vi "Activity Log.vi"(6 "Log File Path":path, 7 "Action":T1, 8 "Error In":errorcluster, 9 "string ref":refnum<vi>, 11 "Message Log Entry":string) -> (0 "Error Out":errorcluster, 3 "Message Log":string)   [LabVIEW 2024]
doc: "This functional global timestamps and records text messages for a generic message log."
uses:
  Activity Log enum Action .ctl
panel:
  in  "Max Lines":i32=8000
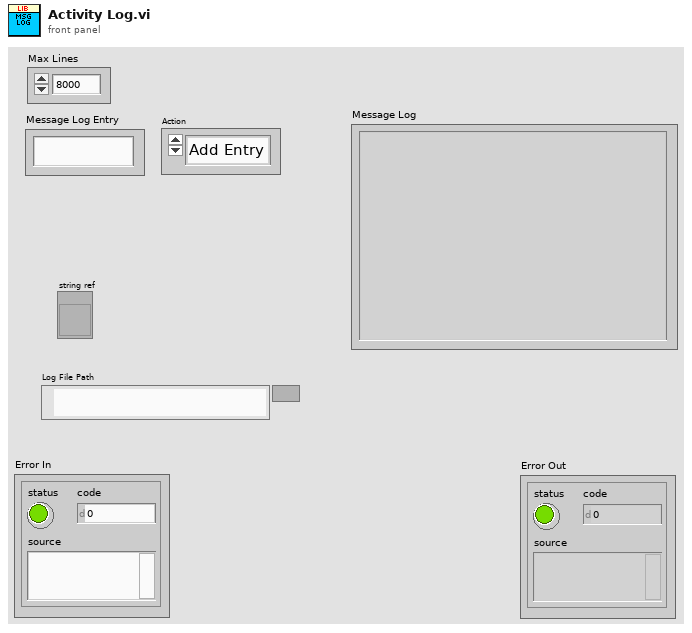
[diagram p1: front panel]
types:
  T1 = typedef "Activity Log enum Action .ctl" = enum16{"Add Entry", "Get Log", "Restore From Disk", "Save to Disk", "Init"}
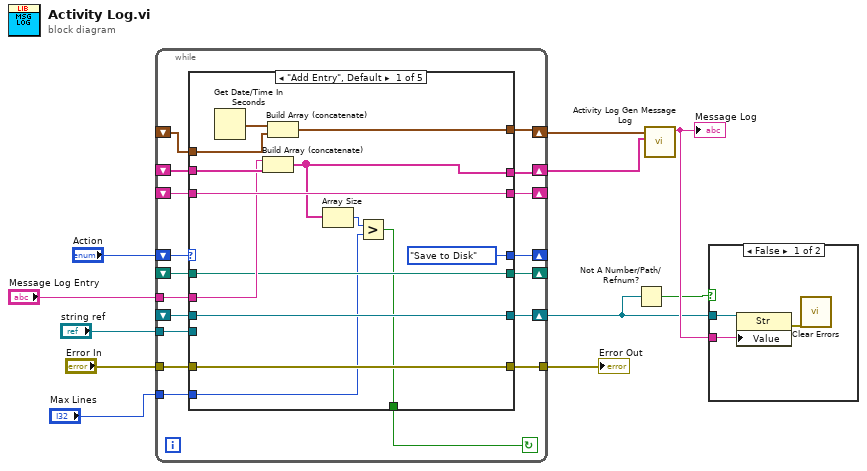
[diagram p0: block diagram]
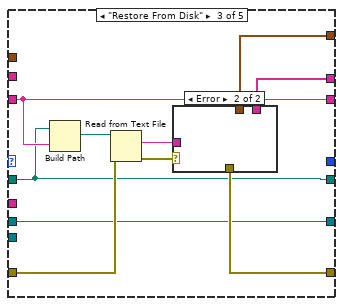
[diagram p4: hidden frame]
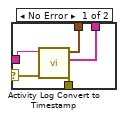
[diagram p5: hidden frame]
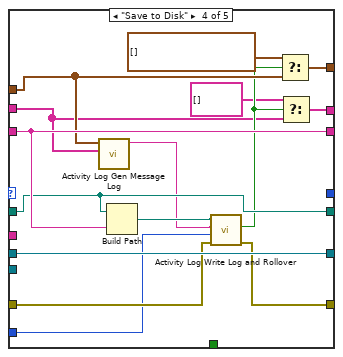
[diagram p6: hidden frame]
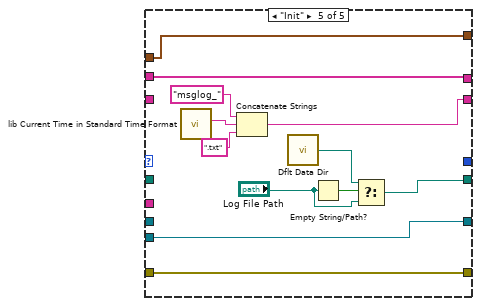
[diagram p7: hidden frame]
diagram:
  n1 = while {
    shift-right: [w26] -> w7
    shift-left: _ -> [w25]
    shift-right: [w27] -> w6
    shift-left: _ -> [w24]
    tunnel: "Message Log Entry" -> [w28]
    tunnel: "Error In" -> [w23]
    tunnel: [w22] -> w8
    shift-right: [w21] -> _
    shift-left: _ -> [w20]
    shift-right: [w19] -> w3
    shift-left: _ -> [w17]
    tunnel: "string ref" -> [w18]
    shift-right: [w16] -> _
    shift-left: _ -> [w15]
    tunnel: "Max Lines" -> [w14]
    shift-right: [w12] -> _
    shift-left: "Action" -> [w29]
    stop <- w13 continue-if-true
    n2 = case shown="\"Add Entry\", Default" w29 {
      tunnel: w28 -> [w39 _ _ _ _]
      tunnel: [w30 w49 w54 w67 w89] -> w27
      tunnel: [w35 w48 w55 w70 w91] -> w26
      tunnel: w25 -> [w38 w48 _ w72 w91]
      tunnel: w24 -> [w43 w49 _ w68 w89]
      tunnel: w23 -> [w42 w47 w57 w76 w90]
      tunnel: [w42 w47 w56 w75 w90] -> w22
      tunnel: [w41 w46 w53 w79 w80] -> w21
      tunnel: w20 -> [w41 w46 w53 w79 _]
      tunnel: [w40 w45 w52 w78 w88] -> w19
      tunnel: w18 -> [_ _ _ _ w88]
      tunnel: w17 -> [w40 w45 w52 w78 _]
      tunnel: [w36 w44 w51 w77 w84] -> w16
      tunnel: w15 -> [w36 w44 w51 w77 _]
      tunnel: w14 -> [w33 _ _ w65 _]
      tunnel: [w32 _ _ _ _] -> w13
      tunnel: [Activity_Log_enum_Action_."Save to Disk" ("Action") _ _ _ _] -> w12
      frame "Add Entry", Default {
        n3 = Get Date/Time In Seconds() -> (seconds since 1Jan1904=w37:timestamp)
        n4 = Build Array (concatenate)(w39, w43) -> (w30:string[])
        n5 = Build Array (concatenate)(w37, w38) -> (w35:timestamp[])
        n6 = Array Size(array=w30) -> (size(s)=w34:i32)
        n7 = Greater?(x=w34, y=w33) -> (0:w32:bool)
      }
      frame "Get Log" {
      }
      frame "Restore From Disk" {
        n8 = Build Path(base path=w51, name or relative path=w53) -> (appended path=w59:path)
        n9 = Read from Text File(file (use dialog)=w59, error in=w57) -> (text=w58:string, error out=w50:errorcluster)  [unwired: 2 in, 2 out]
        n10 = case shown="Error" w50 {
          selector: w50 -> [w60 _]
          tunnel: w58 -> [w64 _]
          tunnel: [w63 _] -> w56
          tunnel: [w62 _] -> w55
          tunnel: [w61 _] -> w54
          frame No Error {
            n11 = call "Activity Log Convert to Timestamp.vi"("error in (no error)"=w60, "Message Log"=w64) -> ("error out"=w63:errorcluster, "Messages"=w61:string[], "timestamps"=w62:timestamp[])  [unwired: 7 in]
          }
          frame Error {
          }
        }
      }
      frame "Save to Disk" {
        n12 = call "Activity Log Gen Message Log.vi"("Messages"=w68, "Timestamps"=w72) -> ("Message Log"=w73:string)  [unwired: 8 in, 1 out]
        n13 = Build Path(base path=w77, name or relative path=w79) -> (appended path=w74:path)
        n14 = call "Activity Log Write Log and Rollover.vi"("error in (no error)"=w76, "Max Size"=w65, "Log Text"=w73, "Log File"=w74) -> ("error out"=w75:errorcluster, "new file?"=w69:bool)  [unwired: 5 in, 1 out]
        n15 = Select(t=timestamp[] [], s=w69, f=w72) -> (s? t:f=w70:timestamp[])
        n16 = Select(t=string[] [], s=w69, f=w68) -> (s? t:f=w67:string[])
      }
      frame "Init" {
        n17 = call "lib Current Time in Standard Time Format.vi"() -> ("date/time string"=w83:string)  [unwired: 11 in]
        n18 = Concatenate Strings("msglog_" ("string"), w83, ".txt" ("string")) -> (w80:string)
        n19 = call <vilib>:"Dflt Data Dir.vi"() -> ("App:Default Data Directory"=w85:path)
        n20 = Empty String/Path?(string/path="Log File Path") -> (empty?=w87:bool)
        n21 = Select(t=w85, s=w87, f="Log File Path") -> (s? t:f=w84:path)
      }
    }
  }
  "Error Out" <- w8
  n22 = Not A Number/Path/Refnum?(number/path/refnum=w3) -> (NaN/Path/Refnum?=w2:bool)
  n23 = call "Activity Log Gen Message Log.vi"("Messages"=w6, "Timestamps"=w7) -> ("Message Log"=w4:string)  [unwired: 8 in, 1 out]
  "Message Log" <- w4
  n24 = case shown="False" w2 {
    tunnel: w4 -> [w94 _]
    tunnel: w3 -> [w93 _]
    frame False {
      n25 = property class="Str"(reference=w93, "Value"=w94) -> (error out=w92:errorcluster)  [unwired: 1 in, 1 out]
      n26 = call <vilib>:"Clear Errors.vi"("error in (no error)"=w92) -> ()  [unwired: 5 in, 2 out]
    }
    frame True {
    }
  }
